vi "3DView.vi"() -> ()   [LabVIEW 2014]
doc: "Use this template to build a VI to use as a subVI."
uses:
  <vilib>/vision/NI_Vision_Development_Module.lvlib
panel:
  out "Dst":T1(plugin-control)
  # ":: MVi Framework V1.0 ::\nAuthor:Gaoke Yang\nEmail: gaoke.yang@yahoo.com\nWeb: www.mvicontrol.com\nCopyright (C) 2015, MVI Technologies All Rights Reserved"
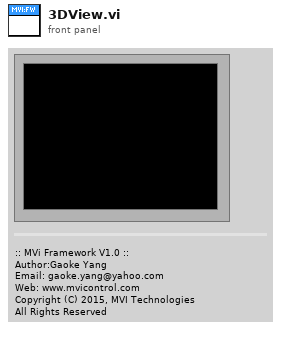
[diagram p1: front panel]
types:
  T1 = typedef "IMAQ Image.ctl" = refnum<image>
  T2 = cluster{"alpha":sgl, "beta":sgl, "border":i32, "background":i32, "plane":i32}
  T3 = enum32{"North West", "South West", "South East", "North East"}
  T4 = typedef "Image Type" = u32
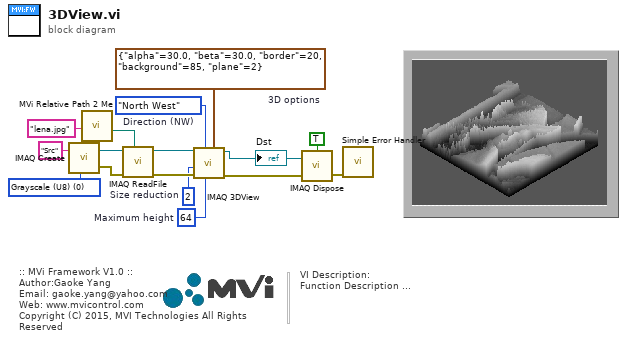
[diagram p0: block diagram]
diagram:
  w1 = T2 {"alpha"=30.0, "beta"=30.0, "border"=20, "background"=85, "plane"=2}  # 3D options
  w2 = T3."North West"  # Direction (NW)
  w3 = 2  # Size reduction
  w4 = 64  # Maximum height
  w9 = T4 0 items=["Grayscale (U8)", "Grayscale (I16)", "Grayscale (SGL)", "Complex (CSG)", "RGB (U32)", "HSL (U32)", "RGB (U64)", "Grayscale (U16)"] ("Image Type")
  # "VI Description:\nFunction Description ..."
  # ":: MVi Framework V1.0 ::\nAuthor:Gaoke Yang\nEmail: gaoke.yang@yahoo.com\nWeb: www.mvicontrol.com\nCopyright (C) 2015, MVI Technologies All Rights Reserved"
  n1 = call "IMAQ Create"("Image Name"="Src" ("name or relative path"), "Image Type"=w9) -> ("New Image"=w11:T1, "error out"=w10:errorcluster)  [unwired: 2 in, 1 out]
  n2 = call "MVi Relative Path 2 Me.vi"("Relative Path"="lena.jpg" ("name or relative path")) -> ("Appended Dir"=w12:path)  [unwired: 5 in, 1 out]
  n3 = call "IMAQ ReadFile"("File Path"=w12, "error in (no error)"=w10, "Image"=w11) -> ("error out"=w8:errorcluster, "Image Out"=w7:T1)  [unwired: 4 in, 3 out]
  n4 = call "IMAQ 3DView"("3D options"=w1, "Maximum height"=w4, "Direction (NW)"=w2, "error in (no error)"=w8, "Size reduction"=w3, "Image Src"=w7) -> ("error out"=w6:errorcluster, "Image Dst Out"=w5:T1)  [unwired: 4 in]
  "Dst" <- w5
  n5 = call "IMAQ Dispose"("All Images? (No)"=TRUE, "Image"=w5, "error in (no error)"=w6) -> ("error out"=w13:errorcluster)  [unwired: 3 out]
  n6 = call <vilib>:"Simple Error Handler.vi"("error in (no error)"=w13) -> ()  [unwired: 1 in, 8 out]
